vi "_Object Tester.vi"() -> ()   [LabVIEW 2025, in "Motor.lvlib" / "Stepper.lvclass"]
uses:
  Stepper.lvclass
  Motor Selection.ctl
  USB IO/Classes/USB-6000/USB-6000.lvclass
  CL57RS/CL57RS.lvclass
  C:/Users/Tyson.Grover/Desktop/Repositories/dqmh-lvoop-template/Libraries/Motor/Classes/Stepper/Stepper.lvclass
  <vilib>/Handler Framework/CmdQueue/Enqueue Single.vi
  Stepper.lvclass/Stepper.ctl
  <vilib>/Handler Framework/Handler Framework.lvlib
panel:
  out "error out":errorcluster
  in  "Tab Control":enum32{"JOG", "Page 2"}(tab)
  in  "Motor Brake":bool
  in  "Clear Motor Error":bool
  in  "CCW?":bool
  in  "JOG":bool
  in  "Speed [rpm]":dbl(slide)=9.818181818181818 min=0.0 max=100.0 scale=0.0..100.0
  in  "Angle":dbl(knob) scale=-180.0..180.0
  in  "Go To Angle":bool
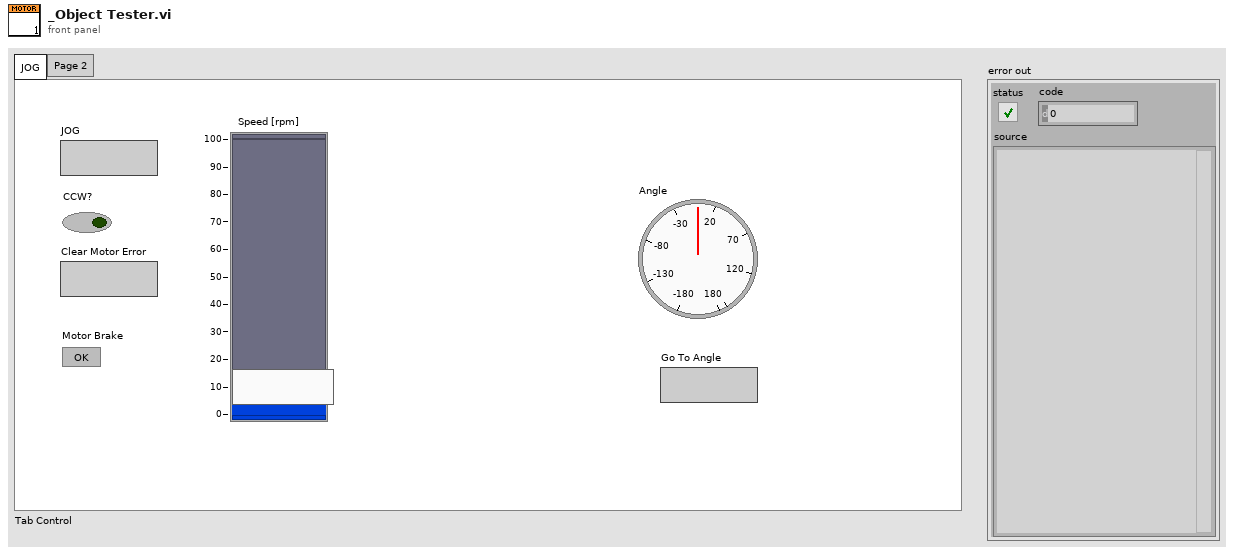
[diagram p1: front panel]
types:
  T1 = typedef "Motor Selection.ctl" = enum16{"Stepper", "CL57RS"}
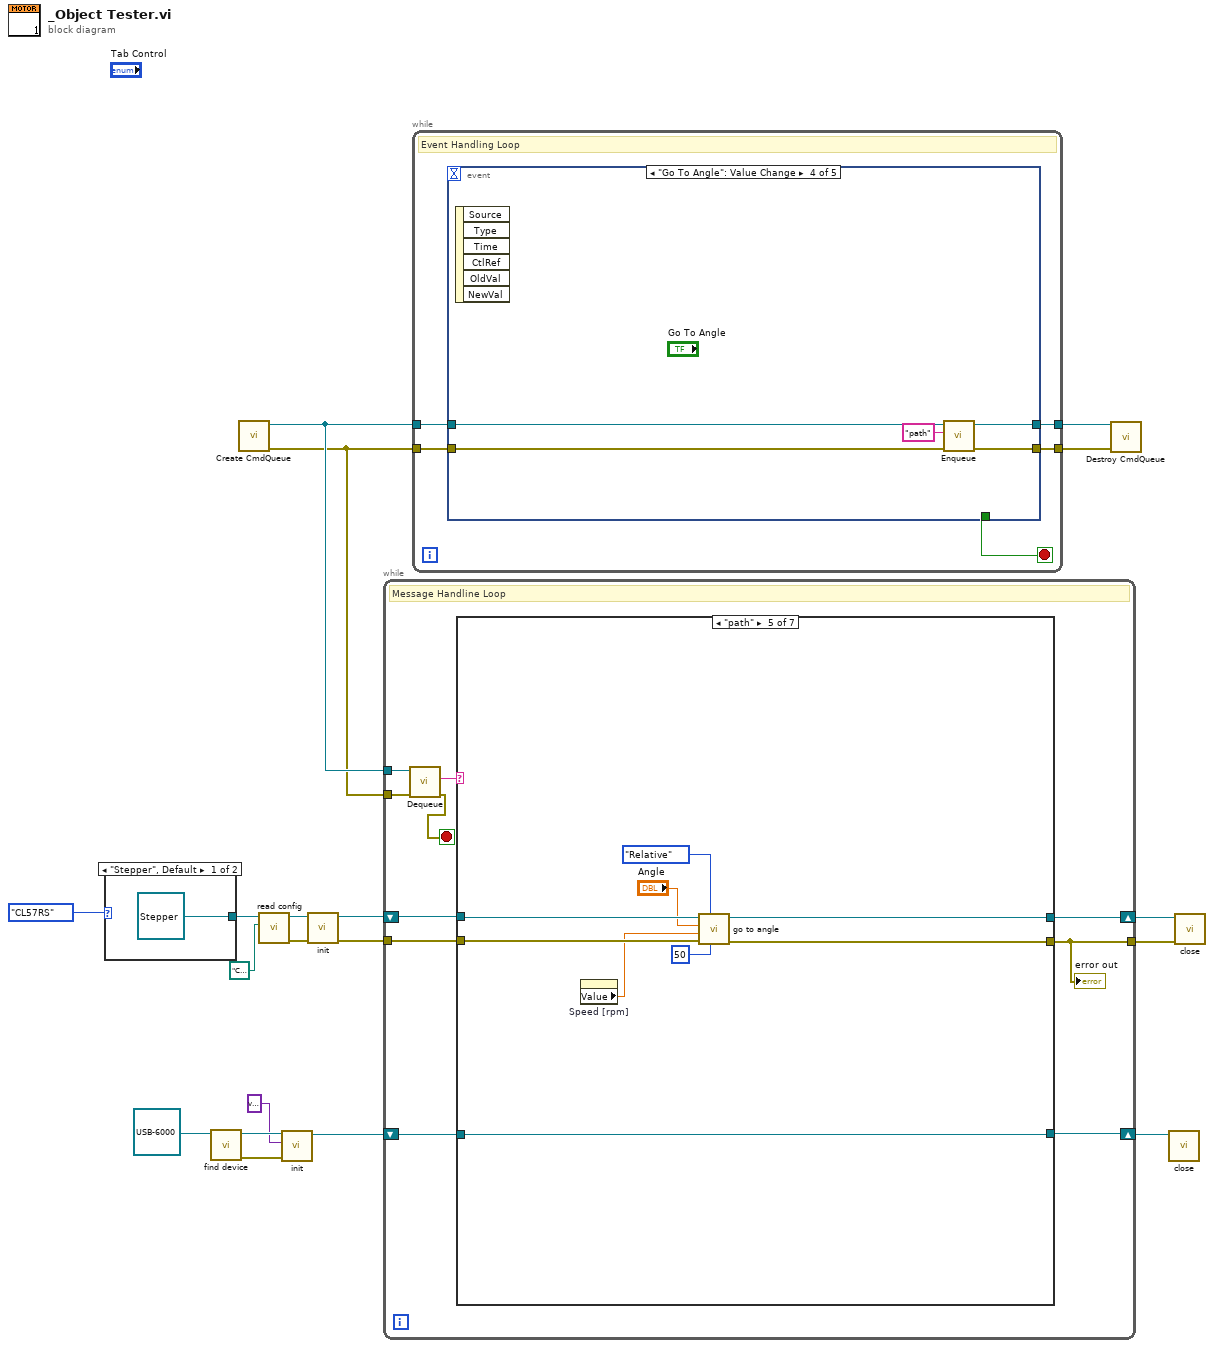
[diagram p0: block diagram]
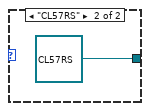
[diagram p2: hidden frame]
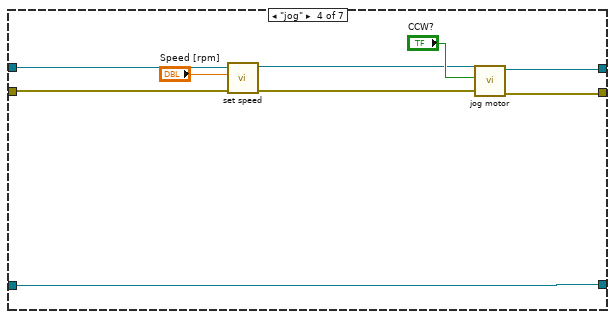
[diagram p6: hidden frame]
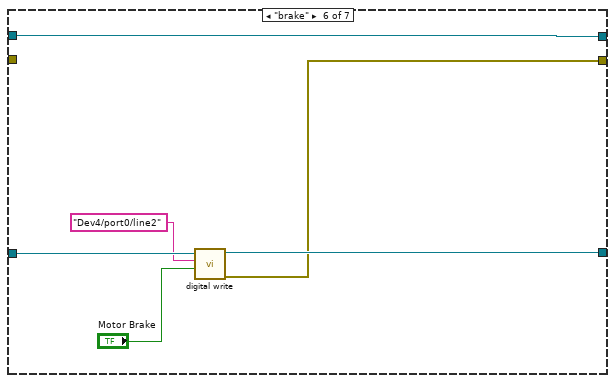
[diagram p7: hidden frame]
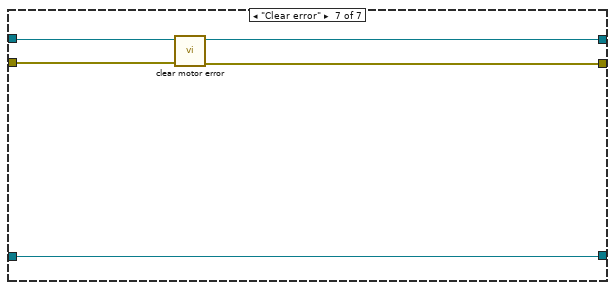
[diagram p8: hidden frame]
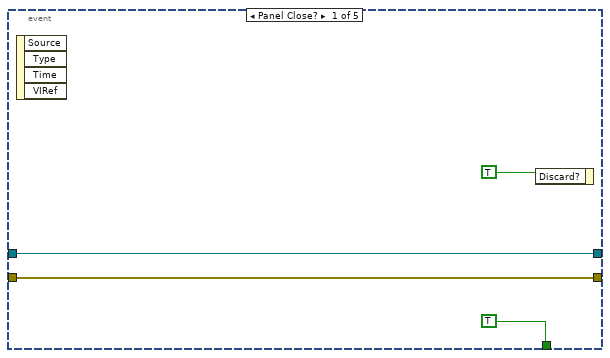
[diagram p9: hidden frame]
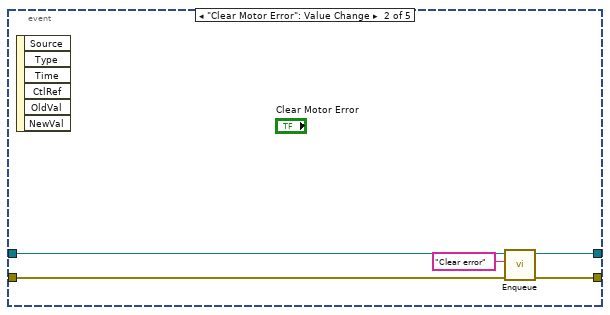
[diagram p10: hidden frame]
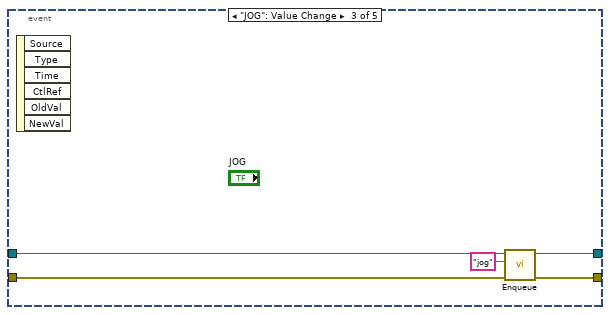
[diagram p11: hidden frame]
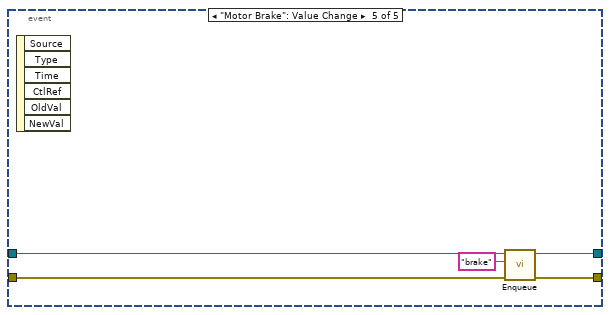
[diagram p12: hidden frame]
diagram:
  n1 = case shown="\"Stepper\", Default" Motor_Selection."CL57RS" {
    tunnel: [refnum<class "Stepper.lvclass"> refnum ("Motor.lvlib:Stepper.lvclass") refnum<class "CL57RS.lvclass"> refnum ("Motor.lvlib:CL57RS.lvclass")] -> w14
    frame "Stepper", Default {
    }
    frame "CL57RS" {
    }
  }
  n2 = call-dynamic "find device.vi"("USB-6000 in"=refnum<class "USB-6000.lvclass"> refnum ("USB IO.lvlib:USB-6000.lvclass")) -> ("error out"=w3:errorcluster, "USB-6000 out"=w5:refnum<class "USB-6000.lvclass">)  [unwired: 9 in]
  n3 = call <vilib>:"Create CmdQueue.vi"() -> ("error out"=w18:errorcluster, "CmdQueue out"=w19:refnum<queue>)  [unwired: 10 in]
  n4 = call-dynamic "read config.vi"("Config File Path"=path "C:/Users/Tyson.Grover/Desktop/Repositories/dqmh-lvoop-template/Config/dqmh-lvoop-template/motor-config.json", "Stepper in"=w14) -> ("error out"=w12:errorcluster, "Stepper out"=w13:refnum<class "Stepper.lvclass">)  [unwired: 8 in]
  n5 = call-dynamic "init.vi"("error in (no error)"=w3, "Variant"=variant, "USB-6000 in"=w5) -> ("USB-6000 out"=w2:refnum<class "USB-6000.lvclass">)  [unwired: 7 in, 1 out]
  n6 = call-dynamic "init.vi"("error in (no error)"=w12, "Stepper in"=w13) -> ("error out"=w9:errorcluster, "Stepper out"=w10:refnum<class "Stepper.lvclass">)  [unwired: 8 in]
  n7 = while {
    tunnel: w19 -> [w31]
    tunnel: w18 -> [w30]
    tunnel: w9 -> [w26]
    shift-right: [w25] -> w8
    shift-left: w10 -> [w27]
    tunnel: [w24] -> w7
    shift-right: [w22] -> w1
    shift-left: w2 -> [w23]
    stop <- w29 stop-if-true
    # "Message Handline Loop"
    n8 = call <vilib>:"Dequeue.vi"("error in (no error)"=w30, "CmdQueue in"=w31) -> ("error out"=w29:errorcluster, "cmd"=w28:string)  [unwired: 5 in, 3 out]
    n9 = case shown="\"path\"" w28 {
      tunnel: w27 -> [w33 w35 w37 w43 w55 w61 w66]
      tunnel: w26 -> [_ _ _ w42 w54 _ w65]
      tunnel: [w33 w35 w37 w46 w52 w61 w64] -> w25
      tunnel: [_ _ _ w45 w53 w56 w63] -> w24
      tunnel: w23 -> [w32 w34 w36 w38 w51 w60 w62]
      tunnel: [w32 w34 w36 w38 w51 w59 w62] -> w22
      frame Default {
      }
      frame "init" {
      }
      frame "shutdown" {
      }
      frame "jog" {
        n10 = call-dynamic "set speed.vi"("error in (no error)"=w42, "Speed [rpm]"="Speed [rpm]", "Stepper in"=w43) -> ("error out"=w40:errorcluster, "Stepper out"=w41:refnum<class "Stepper.lvclass">)  [unwired: 7 in]
        n11 = call-dynamic "jog motor.vi"("error in (no error)"=w40, "CCW? (T)"="CCW?", "Stepper in"=w41) -> ("error out"=w45:errorcluster, "Stepper out"=w46:refnum<class "Stepper.lvclass">)  [unwired: 7 in]
      }
      frame "path" {
        n12 = property on="Speed [rpm]" class="Slide (strict)"() -> ("Value"=w49:dbl)  [unwired: 2 in, 2 out]
        n13 = call-dynamic "go to angle.vi"("Pause Time [ms]"=50, "Relative?"=enum16{"Relative", "Absolute"}."Relative", "error in (no error)"=w54, "Velocity [rpm]"=w49, "Angle"="Angle", "Stepper in"=w55) -> ("error out"=w53:errorcluster, "Stepper out"=w52:refnum<class "Stepper.lvclass">)  [unwired: 4 in]
      }
      frame "brake" {
        n14 = call-dynamic "digital write.vi"("On/Off"="Motor Brake", "Line"="Dev4/port0/line2", "USB-6000 in"=w60) -> ("error out"=w56:errorcluster, "USB-6000 out"=w59:refnum<class "USB-6000.lvclass">)  [unwired: 7 in]
      }
      frame "Clear error" {
        n15 = call-dynamic "clear motor error.vi"("error in (no error)"=w65, "Stepper in"=w66) -> ("error out"=w63:errorcluster, "Stepper out"=w64:refnum<class "Stepper.lvclass">)  [unwired: 8 in]
      }
    }
    "error out" <- w24
  }
  n16 = while {
    tunnel: w19 -> [w70]
    tunnel: w18 -> [w69]
    tunnel: [w68] -> w17
    tunnel: [w67] -> w16
    stop <- w71 stop-if-true
    # "Event Handling Loop"
    n17 = event shown="[3] \"Go To Angle\": Value Change" {
      selector: _ -> [_ _ _ _ _]
      dyn-events: _ -> [_ _ _ _ _]
      timeout: _ -> [_ _ _ _ _]
      tunnel: [TRUE _ _ _ _] -> w71
      tunnel: w70 -> [w73 w77 w82 w87 w92]
      tunnel: w69 -> [w72 w78 w83 w88 w93]
      tunnel: [w73 w80 w85 w90 w95] -> w68
      tunnel: [w72 w79 w84 w89 w94] -> w67
      event Panel Close? {
        n18 = event-data() -> ()  [unwired: 1 in, 4 out]
        n19 = event-data("Discard?"=TRUE) -> ()  [unwired: 1 in, 1 out]
      }
      event "Clear Motor Error": Value Change {
        n20 = event-data() -> ()  [unwired: 1 in, 6 out]
        n21 = call-poly <vilib>:"Enqueue.vi"("error in (no error)"=w78, "Command"="Clear error", "CmdQueue in"=w77) -> ("error out"=w79:errorcluster, "CmdQueue out"=w80:refnum<queue>)  [unwired: 7 in]
      }
      event "JOG": Value Change {
        n22 = event-data() -> ()  [unwired: 1 in, 6 out]
        n23 = call-poly <vilib>:"Enqueue.vi"("error in (no error)"=w83, "Command"="jog", "CmdQueue in"=w82) -> ("error out"=w84:errorcluster, "CmdQueue out"=w85:refnum<queue>)  [unwired: 7 in]
      }
      event "Go To Angle": Value Change {
        n24 = event-data() -> ()  [unwired: 1 in, 6 out]
        n25 = call-poly <vilib>:"Enqueue.vi"("error in (no error)"=w88, "Command"="path", "CmdQueue in"=w87) -> ("error out"=w89:errorcluster, "CmdQueue out"=w90:refnum<queue>)  [unwired: 7 in]
      }
      event "Motor Brake": Value Change {
        n26 = event-data() -> ()  [unwired: 1 in, 6 out]
        n27 = call-poly <vilib>:"Enqueue.vi"("error in (no error)"=w93, "Command"="brake", "CmdQueue in"=w92) -> ("error out"=w94:errorcluster, "CmdQueue out"=w95:refnum<queue>)  [unwired: 7 in]
      }
    }
  }
  n28 = call <vilib>:"Destroy CmdQueue.vi"("error in (no error)"=w16, "CmdQueue in"=w17) -> ()  [unwired: 9 in, 1 out]
  n29 = call-dynamic "close.vi"("USB-6000 in"=w1) -> ()  [unwired: 9 in, 2 out]
  n30 = call-dynamic "close.vi"("error in (no error)"=w7, "Stepper in"=w8) -> ()  [unwired: 8 in, 2 out]
